vi "Finish.vi"(8 "error in (no error)":errorcluster, 11 "Solenoids in":refnum<class "Solenoids.lvclass">) -> (0 "error out":errorcluster, 3 "Solenoids out":refnum<class "Solenoids.lvclass">)   [LabVIEW 2018, in "Pneumatics control.lvlib" / "Solenoids.lvclass"]
doc: "It takes a RefNum and closes the solonoid."
uses:
  Solenoids.lvclass
  Solenoids.lvclass/Solenoids.ctl
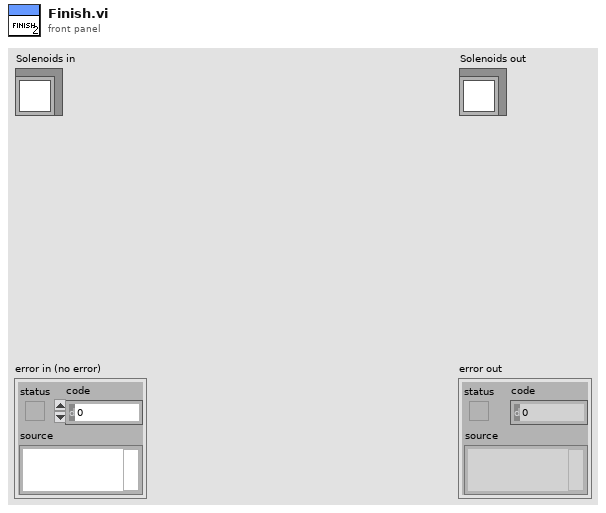
[diagram p1: front panel]
types:
  T1 = typedef "WPI_SolenoidDevRef.ctl" = cluster{"DevStatus":errorcluster, "Pneumatics Control Module":u8, "Forward Solenoid Channel":T2, "Reverse Solenoid Channel":T2}
  T2 = typedef "WPI_SolenoidChannel.ctl" = enum8{"Solenoid 0", "Solenoid 1", "Solenoid 2", "Solenoid 3", "Solenoid 4", "Solenoid 5", "Solenoid 6", "Solenoid 7", "Invalid"}
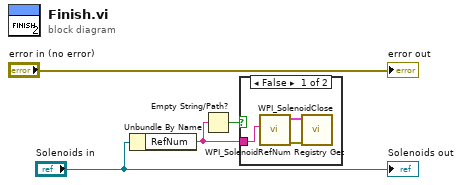
[diagram p0: block diagram]
diagram:
  n1 = Unbundle By Name("Solenoids in") -> ("RefNum"=w2:string)
  n2 = Empty String/Path?(string/path=w2) -> (empty?=w1:bool)
  n3 = case shown="False" w1 {
    tunnel: w2 -> [w5 _]
    frame False {
      n4 = call <vilib>:"WPI_SolenoidRefNum Registry Get.vi"("refnum name"=w5) -> ("error out"=w7:errorcluster, "SolenoidDevRef"=w6:T1)  [unwired: 9 in]
      n5 = call <vilib>:"WPI_SolenoidClose.vi"("error in (no error)"=w7, "SolenoidDevRef"=w6) -> ()  [unwired: 9 in, 1 out]
    }
    frame True {
    }
  }
  "error out" <- "error in (no error)"
  "Solenoids out" <- "Solenoids in"
